vi "SRDG535.destructor.vi"(0 "i ref in":refnum<vi>, 5 "error in":errorcluster) -> (19 "error out":errorcluster)   [LabVIEW 2014, in "SRDG535.lvlib"]
doc: "This is the destructor of a class.\n\nLicense Agreement for this software:\n\nCopyright (C)\nGesellschaft für Schwerionenforschung, GSI\nPlanckstr. 1\n64291 Darmstadt\nGermany\n\nContact: D.Beck@gsi.de \n\nThis program is free software; you can redistribute it and/or modify it under the terms of the \nGNU General Public License as published by the Free Software Foundation; either version 2 of \nthe license, or (at your option) any later version.\n\nThis program is distributed in the hope that it will be useful, but WITHOUT ANY WARRANTY; \nwithout even the implied warranty of MERCHANTABILITY or FITNESS FOR A PARTICULAR PURPOSE. See the GNU General License for more details (http://www.gnu.org).\n\nGesellschaft für Schwerionenforschung, GSI\nPlanckstr. 1, 64291 Darmstadt, Germany\nFor all questions and ideas contact: M.Richter@gsi.de, H.Brand@gsi.de or D.Beck@gsi.de.\nLast update: 16-JUN-2004"
uses:
  SRDG535.lvlib
  lib.lib/DimLVEvent/LVDimInterface/LVDimInterface.lvlib
  CSPhelix/PH_PSDBWriter/PH_PSDBWriter.lvlib
  CSPhelix/PH_StatusHandler/PH_StatusHandler.lvlib
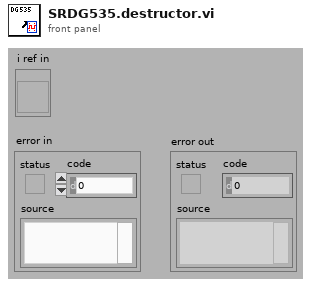
[diagram p1: front panel]
types:
  T1 = typedef "SRDG535.lvlib/SRDG535.i attribute.ctl" = cluster{"GPIB address":string, "Device error":errorcluster, "GUI Refs":cluster{"Delete":refnum<vi>, "Device Error":refnum<vi>, "Information":refnum<vi>, "Output":refnum<vi>, "Delay":refnum<vi>, "Trigger":refnum<vi>}, "Output Settings":T2, "Service ID Rate":i32, "Service IDs Channelinfo":i32[], "Delay Settings":T4, "Trigger Settings":T5}
  T2 = typedef "SRDG535.lvlib/SRDG535.Output.ctl" = cluster{"CH T0":T3, "CH A":T3, "CH B":T3, "CH AB":T3, "CH C":T3, "CH D":T3, "CH CD":T3}
  T3 = typedef "SRDG535.lvlib/SRDG535.Channel Output.ctl" = cluster{"Inversion":bool, "Amplitude (V)":dbl, "Offset (V)":dbl, "Mode":i32, "Load":bool}
  T4 = typedef "SRDG535.lvlib/SRDG535.Delay.ctl" = cluster{"CH A":cluster{"rel to":u32, "Delay (s)":dbl}, "CH B":cluster{"rel to":u32, "Delay (s)":dbl}, "CH C":cluster{"rel to":u32, "Delay (s)":dbl}, "CH D":cluster{"rel to":u32, "Delay (s)":dbl}}
  T5 = typedef "SRDG535.lvlib/SRDG535.Trigger.ctl" = cluster{"trigger":u32, "Impedance":bool, "Slope":bool, "burst count":i32, "external level (V)":sgl, "Internal/Burst Rate (Hz)":dbl, "Burst Period":i32}
  T6 = enum16{"SetAttribute", "GetAttribute", "CreateAttribute", "DestroyAttribute", "DestroyAllAtributes"}
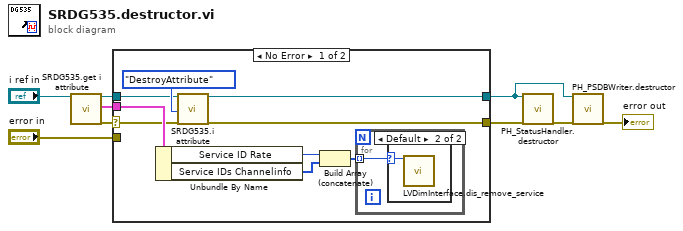
[diagram p0: block diagram]
diagram:
  n1 = call "SRDG535.get i attribute.vi"("i ref in"="i ref in") -> ("i ref out"=w7:refnum<vi>, "i attribute"=w6:T1, "error out"=w2:errorcluster)  [unwired: 16 in]
  n2 = case shown="No Error" w2 {
    selector: w2 -> [w10 _]
    tunnel: [w17 w21] -> w9
    tunnel: w7 -> [w16 w22]
    tunnel: w6 -> [w15 _]
    tunnel: [w11 w22] -> w3
    tunnel: "error in" -> [_ w21]
    frame No Error {
      n3 = Unbundle By Name(w15) -> ("Service ID Rate"=w13:i32, "Service IDs Channelinfo"=w12:i32[])
      n4 = call "SRDG535.i attribute.vi"("VI Refnum"=w16, "Action"=T6."DestroyAttribute", "error in (no error)"=w10) -> ("VI Refnum out"=w11:refnum<vi>, "error out"=w17:errorcluster)  [unwired: 14 in, 1 out]
      n5 = Build Array (concatenate)(w13, w12) -> (w14:i32[])
      n6 = for {
        tunnel: w14 -> [w19] mode=indexing
        n7 = case shown="Default" w19 {
          selector: w19 -> [_ w20]
          frame -1 {
          }
          frame Default {
            n8 = call "LVDimInterface.dis_remove_service.vi"("my_serviceID"=w20) -> ()  [unwired: 18 in, 1 out]
          }
        }
      }
    }
    frame Error {
    }
  }
  n9 = call "PH_StatusHandler.destructor.vi"("i ref in"=w3, "error in(no error)"=w9) -> ("error out"=w4:errorcluster)  [unwired: 17 in]
  n10 = call "PH_PSDBWriter.destructor.vi"("i ref in"=w3, "error in(no error)"=w4) -> ("error out"=→"error out":errorcluster)  [unwired: 17 in]
